vi "cosine_sigmoid.vi"(3 "output control":T1, 4 "data":variant, 5 "X":dbl[](array[numeric]), 6 "a":dbl[](array[numeric])) -> (0 "error out":errorcluster, 1 "f'(X,a)":dbl[][](array[numeric]), 2 "f(X,a)":dbl[](array[numeric]))   [LabVIEW 2019]
doc: "This template is the starting point for creating a model function to be passed to the Nonlinear Curve Fit.vi."
uses:
  <vilib>/gmath/NumericalOptimization/LM_output select.ctl
  <vilib>/gmath/NI_Gmath.lvlib
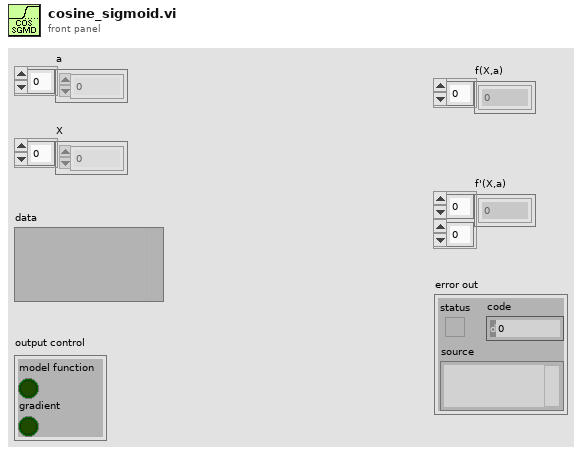
[diagram p1: front panel]
types:
  T1 = typedef "NI_Gmath.lvlib/LM_output select.ctl" = cluster{"model function":bool, "gradient":bool}
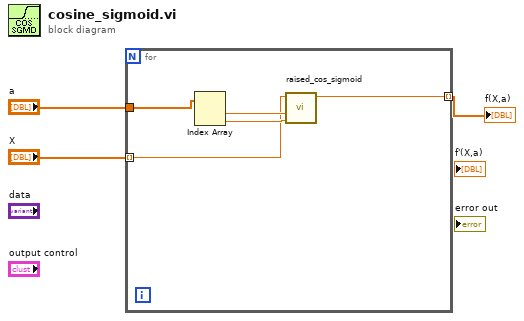
[diagram p0: block diagram]
diagram:
  n1 = for {
    tunnel: "a" -> [w8]
    tunnel: "X" -> [w5] mode=indexing
    tunnel: [w4] -> w1 mode=indexing
    n2 = Index Array(array=w8) -> (element #1=w7:dbl, element #2=w6:dbl)  [unwired: 2 in]
    n3 = call "raised_cos_sigmoid.vi"("B"=w6, "A"=w7, "x"=w5) -> ("raised_cos_sigmoid(x, A, B)"=w4:dbl)  [unwired: 8 in]
  }
  "f(X,a)" <- w1
